vi "Load_app.vi"   [LabVIEW 2025]
uses:
  ATM-Controller/ATM-Controller/ATM-Controller.lvclass
  C:/Program Files (x86)/National Instruments/LabVIEW 2025/vi.lib/ActorFramework/Actor/Actor.lvclass
  <vilib>/ActorFramework/Actor/Actor.lvclass
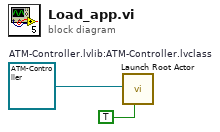
[diagram p0: block diagram]
diagram:
  w2 = refnum<class "ATM-Controller.lvclass"> refnum  # ATM-Controller.lvlib:ATM-Controller.lvclass
  n1 = call <vilib>:"Launch Root Actor.vi"("Open Actor Core front panel? (F)"=TRUE, "Actor"=w2) -> ()  [unwired: 8 in, 2 out]
